vi "EZ1 MB1010 Sonar - Analog.vi"() -> ()   [LabVIEW 2025]
doc: "This example shows how to use the MaxBotix LV-MaxSonar-EZ1 Sonar Range Finder MB1010. It will display the distance from the sensor in inches.\n\nThis example expects a USB cable connected from your development PC to the Type B USB Jack (next to the power input) on the roboRIO."
uses:
  <vilib>/Rock Robotics/SystemInterfaces/AI/FPGA_AIChannel.ctl
  <vilib>/Rock Robotics/WPI/Ultrasonic/WPI_SonarMB1010AnalogOpen.vi
  <vilib>/Rock Robotics/WPI/Ultrasonic/WPI_SonarMB1010AnalogGetRange.vi
  <vilib>/Rock Robotics/WPI/Ultrasonic/WPI_SonarMB1010AnalogClose.vi
panel:
  out "distance":dbl(slide)=125.0 scale=0.0..250.0 scale format="%3d"
  in  "Scaling factor (V/in)":dbl=0.0098
  in  "Average Bits":u8=3 max=15
  in  "Channel":T1=enum."AI 2"
  in  "stop":bool
  # "Set these inputs before running."
  # "EZ1 MB1010\nGND (black wire)------\n+5 (red wire)----------\nAN (white wire)-------"
  # "roboRIO\nAI-2 \nAI-2     V\nAI-2     S"
  # "This shows wiring for a MaxBotix LV-MaxSonar-EZ1 Sonar Range Finder MB1010."
  # "EZ1 MB1010"
  # "GND"
  # "+5"
  # "TX"
  # "RX"
  # "AN"
  # "PW"
  # "BW"
  # "Output information."
  # "EZ1"
  # "inches"
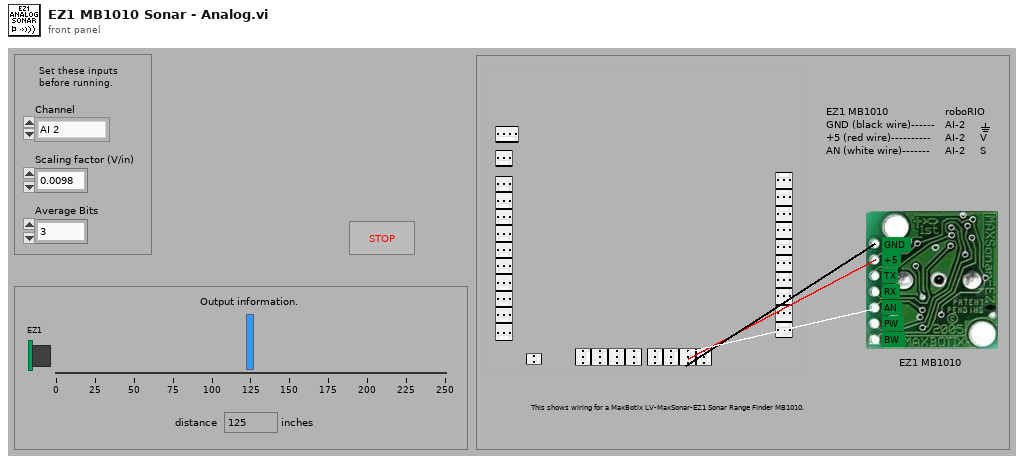
[diagram p1: front panel]
types:
  T1 = typedef "FPGA_AIChannel.ctl" = enum8{"AI 0", "AI 1", "AI 2", "AI 3", "AI MXP 0", "AI MXP 1", "AI MXP 2", "AI MXP 3", "Invalid"}
  T2 = typedef "WPI_SonarMB1010AnalogDeviceRef.ctl" = cluster{"AIDeviceRef":T3, "Scaling factor (V/in)":dbl, "Average Bits":u8}
  T3 = typedef "WPI_AnalogChannelDevRef.ctl" = cluster{"DevStatus":errorcluster, "Analog Channel":T1}
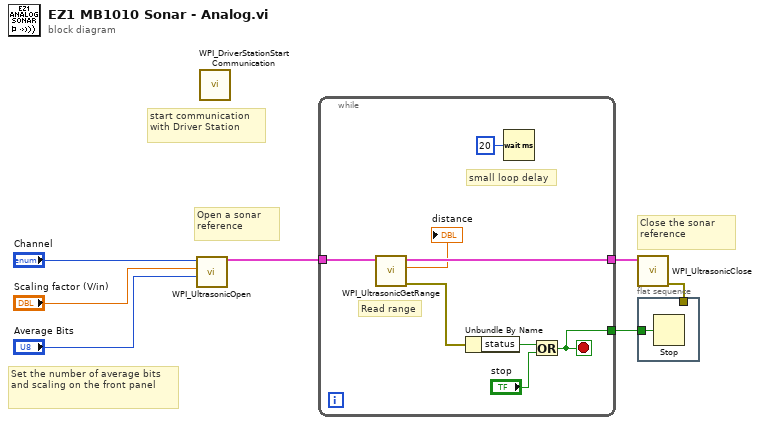
[diagram p0: block diagram]
diagram:
  # "Set the number of average bits and scaling on the front panel"
  # "start communication with Driver Station"
  # "Close the sonar reference"
  # "Open a sonar reference"
  n1 = call-poly <vilib>:"WPI_UltrasonicOpen.vi"("Average Bits"="Average Bits", "Scaling factor (V/in)"="Scaling factor (V/in)", "Analog Channel"="Channel") -> ("SonarMB1010AnalogDevRef"=w5:T2)  [unwired: 7 in, 1 out]
  n2 = call <vilib>:"WPI_DriverStationStart Communication.vi"() -> ()  [unwired: 3 in, 9 out]
  n3 = while {
    tunnel: w5 -> [w9]
    tunnel: [w15] -> w2
    tunnel: [w10] -> w7
    stop <- w10 stop-if-true
    # "small loop delay"
    # "Read range"
    n4 = call-poly <vilib>:"WPI_UltrasonicGetRange.vi"("SonarMB1010AnalogDevRef"=w9) -> ("error out"=w11:errorcluster, "Distance"=→"distance":dbl, "SonarMB1010AnalogDevRef"=w15:T2)  [unwired: 8 in]
    n5 = Unbundle By Name(w11) -> ("status"=w13:bool)
    n6 = Wait (ms)(milliseconds to wait=u32 20) -> ()  [unwired: 1 out]
    n7 = Or(x=w13, y="stop") -> (x .or. y?=w10:bool)
  }
  n8 = call-poly <vilib>:"WPI_UltrasonicClose.vi"("SonarMB1010AnalogDevRef"=w2) -> ("error out"=w1:errorcluster)  [unwired: 10 in]
  n9 = flat-sequence {
    tunnel: w7 -> [w16]
    tunnel: w1 -> [_]
    frame #0 {
      n10 = Stop(stop? (T)=w16) -> ()
    }
  }
